vi "Test Call Skipping Method.vi"(8 "error in (no error)":errorcluster, 11 "Test Case In":refnum<class "Test Case Test.lvclass">) -> (0 "error out":errorcluster, 3 "Test Case Out":refnum<class "Test Case Test.lvclass">)   [LabVIEW 2020, in "Test Case Test.lvclass"]
uses:
  Test Case Test.lvclass
  C:/Program Files (x86)/National Instruments/LabVIEW 2020/vi.lib/Astemes/LUnit/Test Case.lvclass
  source/Core/Result/Status.ctl
  Test Doubles/Test Case Test Double/Methods.ctl
  <vilib>/Astemes/LUnit/Test Case.lvclass/Test Case.ctl
  e8c5eeff-a694-4c0d-b261-74e2e6f5327d.vi
  <vilib>/Astemes/LUnit/Core/LUnit Test Case/Private/Append Pass Result.vi
  <vilib>/Astemes/LUnit/Core/LUnit Test Case/Private/Append Fail Result.vi
  e8c5eeff-a694-4c0d-b261-74e2e6f5327d.vi/9c5d11cd-9439-4240-a1ee-d9baace9c924.vi
  <vilib>/Astemes/LUnit/Core/LUnit Test Case/Private/Run In UI.vi
  <vilib>/Utility/error.llb/Clear Errors.vi
  source/LUnit Test Case.lvclass
  source/Core/Result/Result.lvlib
  Test Doubles/Test Case Test Double/Test Case Test Double.lvclass
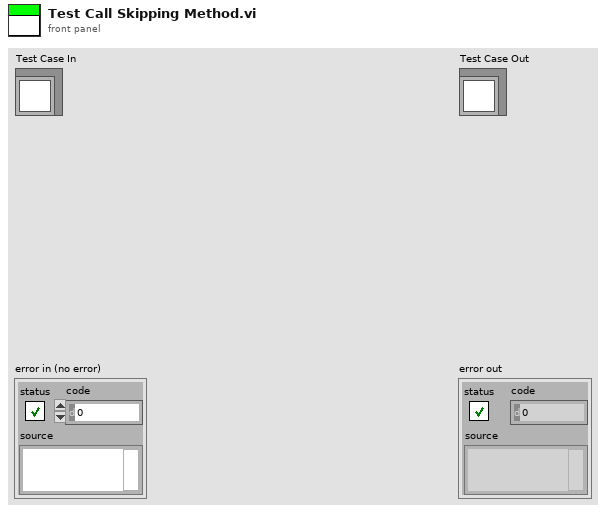
[diagram p1: front panel]
types:
  T1 = typedef "Test Case Test Double.lvclass/Methods.ctl" = enum16{"Test Failing Test.vi", "Test Passing Test.vi", "Test Error Test.vi", "Test Skip Test.vi", "Test Passing Pass If Test.vi", "Test Failing Pass If Test.vi", "Test Failing Fail If Test.vi", "Test Passing Fail If Test.vi", "Test Passing Pass If Error Test.vi", "Test Failing Pass If Error Test.vi", "Test Passing Fail If Error Test.vi", "Test Failing Fail If Error Test.vi", "Test Passing Pass If Equal Test.vi", "Test Failing Pass If Equal Test.vi", "Test Failing Fail If Equal Test.vi", "Test Passing Fail If Equal Test.vi", "Freezing Test.vi", "Test Pass on Expected Error Code.vi", "Test Error on Unexpected Error Code.vi", "Test Fail on Expected Error Code.vi", "Test Error when Fail on Unexpected Error Code.vi", "Test Pass on Expected Element in Array.vi", "Test Fail on Expected Element Not in Array.vi", "Test Pass on Expected Element in Set.vi", "Test Fail on Expected Element Not in Set.vi", "Test Pass on Expected Element in Map.vi", "Test Fail on Expected Element Not in Map.vi", "Test Fail on Unexpected Element in Array.vi", "Test Pass on Unexpected Element Not in Array.vi", "Test Fail if Unexpected Element in Set.vi", "Test Pass if Unexpected Element Not in Set.vi", "Test Fail if Unexpected Element in Map.vi", "Test Pass if Unexpected Element Not in Map.vi", "Test Pass on Expected Element in Array of Clusters.vi", "Test Pass on Expected Element Not in Array of Clusters.vi", "Test Matching String Test.vi", "Test Not Matching String Test.vi", "Verify Passing.vi", "Without Prefix.vi", "Private VI.vi"}
  T2 = typedef "Result.lvlib/Status.ctl" = enum16{"", "Passed", "Failed", "Error", "Skipped", "Setup Error", "Broken", "Teardown Error"}
  T3 = typedef "Result.lvlib/Result.ctl" = cluster{"Name":string, "Description":string, "Status":T2, "Result Type":T4, "Execution Time":dbl, "Data":cluster{"Expected":variant, "Actual":variant, "Delta":variant}}
  T4 = typedef "Result.lvlib/Type.ctl" = enum16{"Test Case", "Test Suite", "Test Run", "Pass", "Fail", "Skip", "Pass if", "Fail if", "Pass if Error", "Fail if Error", "Pass if Equal", "Fail if Equal"}
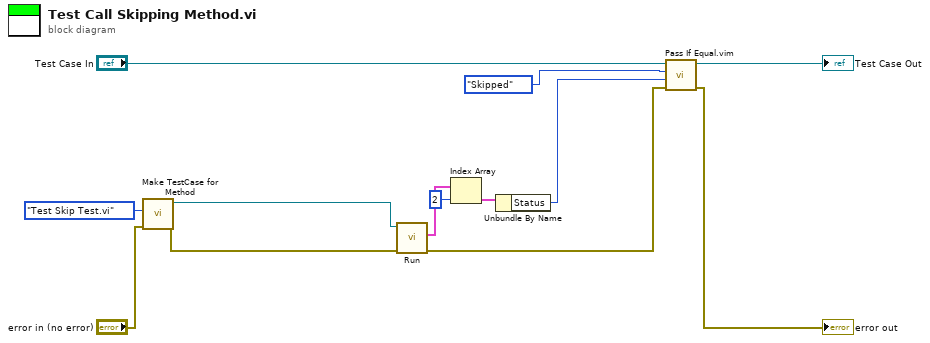
[diagram p0: block diagram]
diagram:
  n1 = call "Make TestCase for Method.vi"("error in (no error)"="error in (no error)", "Test Method"=Methods."Test Skip Test.vi") -> ("error out"=w9:errorcluster, "LUnit Test Case V2 out"=w10:refnum<class "LUnit Test Case.lvclass">)  [unwired: 8 in]
  n2 = call-dynamic "Run.vi"("error in (no error)"=w9, "LUnit Test Case In"=w10) -> ("error out"=w7:errorcluster, "Results"=w6:T3[])  [unwired: 6 in, 2 out]
  n3 = Index Array(array=w6, index=2) -> (element=w5:T3)
  n4 = Unbundle By Name(w5) -> ("Status"=w4:T2)
  n5 = call "Pass If Equal.vim"("error in (no error)"=w7, "Actual"=w4, "Expected"=Status."Skipped" ("Status"), "LUnit Test Case In"="Test Case In") -> ("error out"=→"error out":errorcluster, "LUnit Test Case Out"=→"Test Case Out":refnum<class "Test Case Test.lvclass">)  [unwired: 6 in]
